vi "ModuloTeste.vi"(0 "IA State Input":T3 {"enemy_robots"."Agentes Disponíveis" format="%#_13g"; "our_robots"."Agentes Disponíveis" format="%#_13g"}, 1 "atacando ao contrário?":bool=TRUE, 3 "test module":T1) -> (14 "IA State Output":T3 {"enemy_robots"."Agentes Disponíveis" format="%#_13g"; "our_robots"."Agentes Disponíveis" format="%#_13g"}, 15 "ball":dbl(graph), 17 "Robot":dbl(graph))   [LabVIEW 2018]
uses:
  Core/AI Input.ctl
  Core/AI Robot.ctl
  Functions Enum.ctl
  AttackerStates.ctl
  Path Planning/RRT/PathDests.ctl
  Path Planning/RRT/PathDest.ctl
  Core/AI Ball.ctl
  Core/Field Size.ctl
  Core/AI Judge.ctl
  Command Enum.ctl
  Util/Events/Events.ctl
  Test/TestModule.ctl
  Util/Select None or Robot.ctl
  <vilib>/Analysis/_algsub.llb/Real Vector Norm.vi
  <vilib>/Analysis/NI_AALPro.lvlib
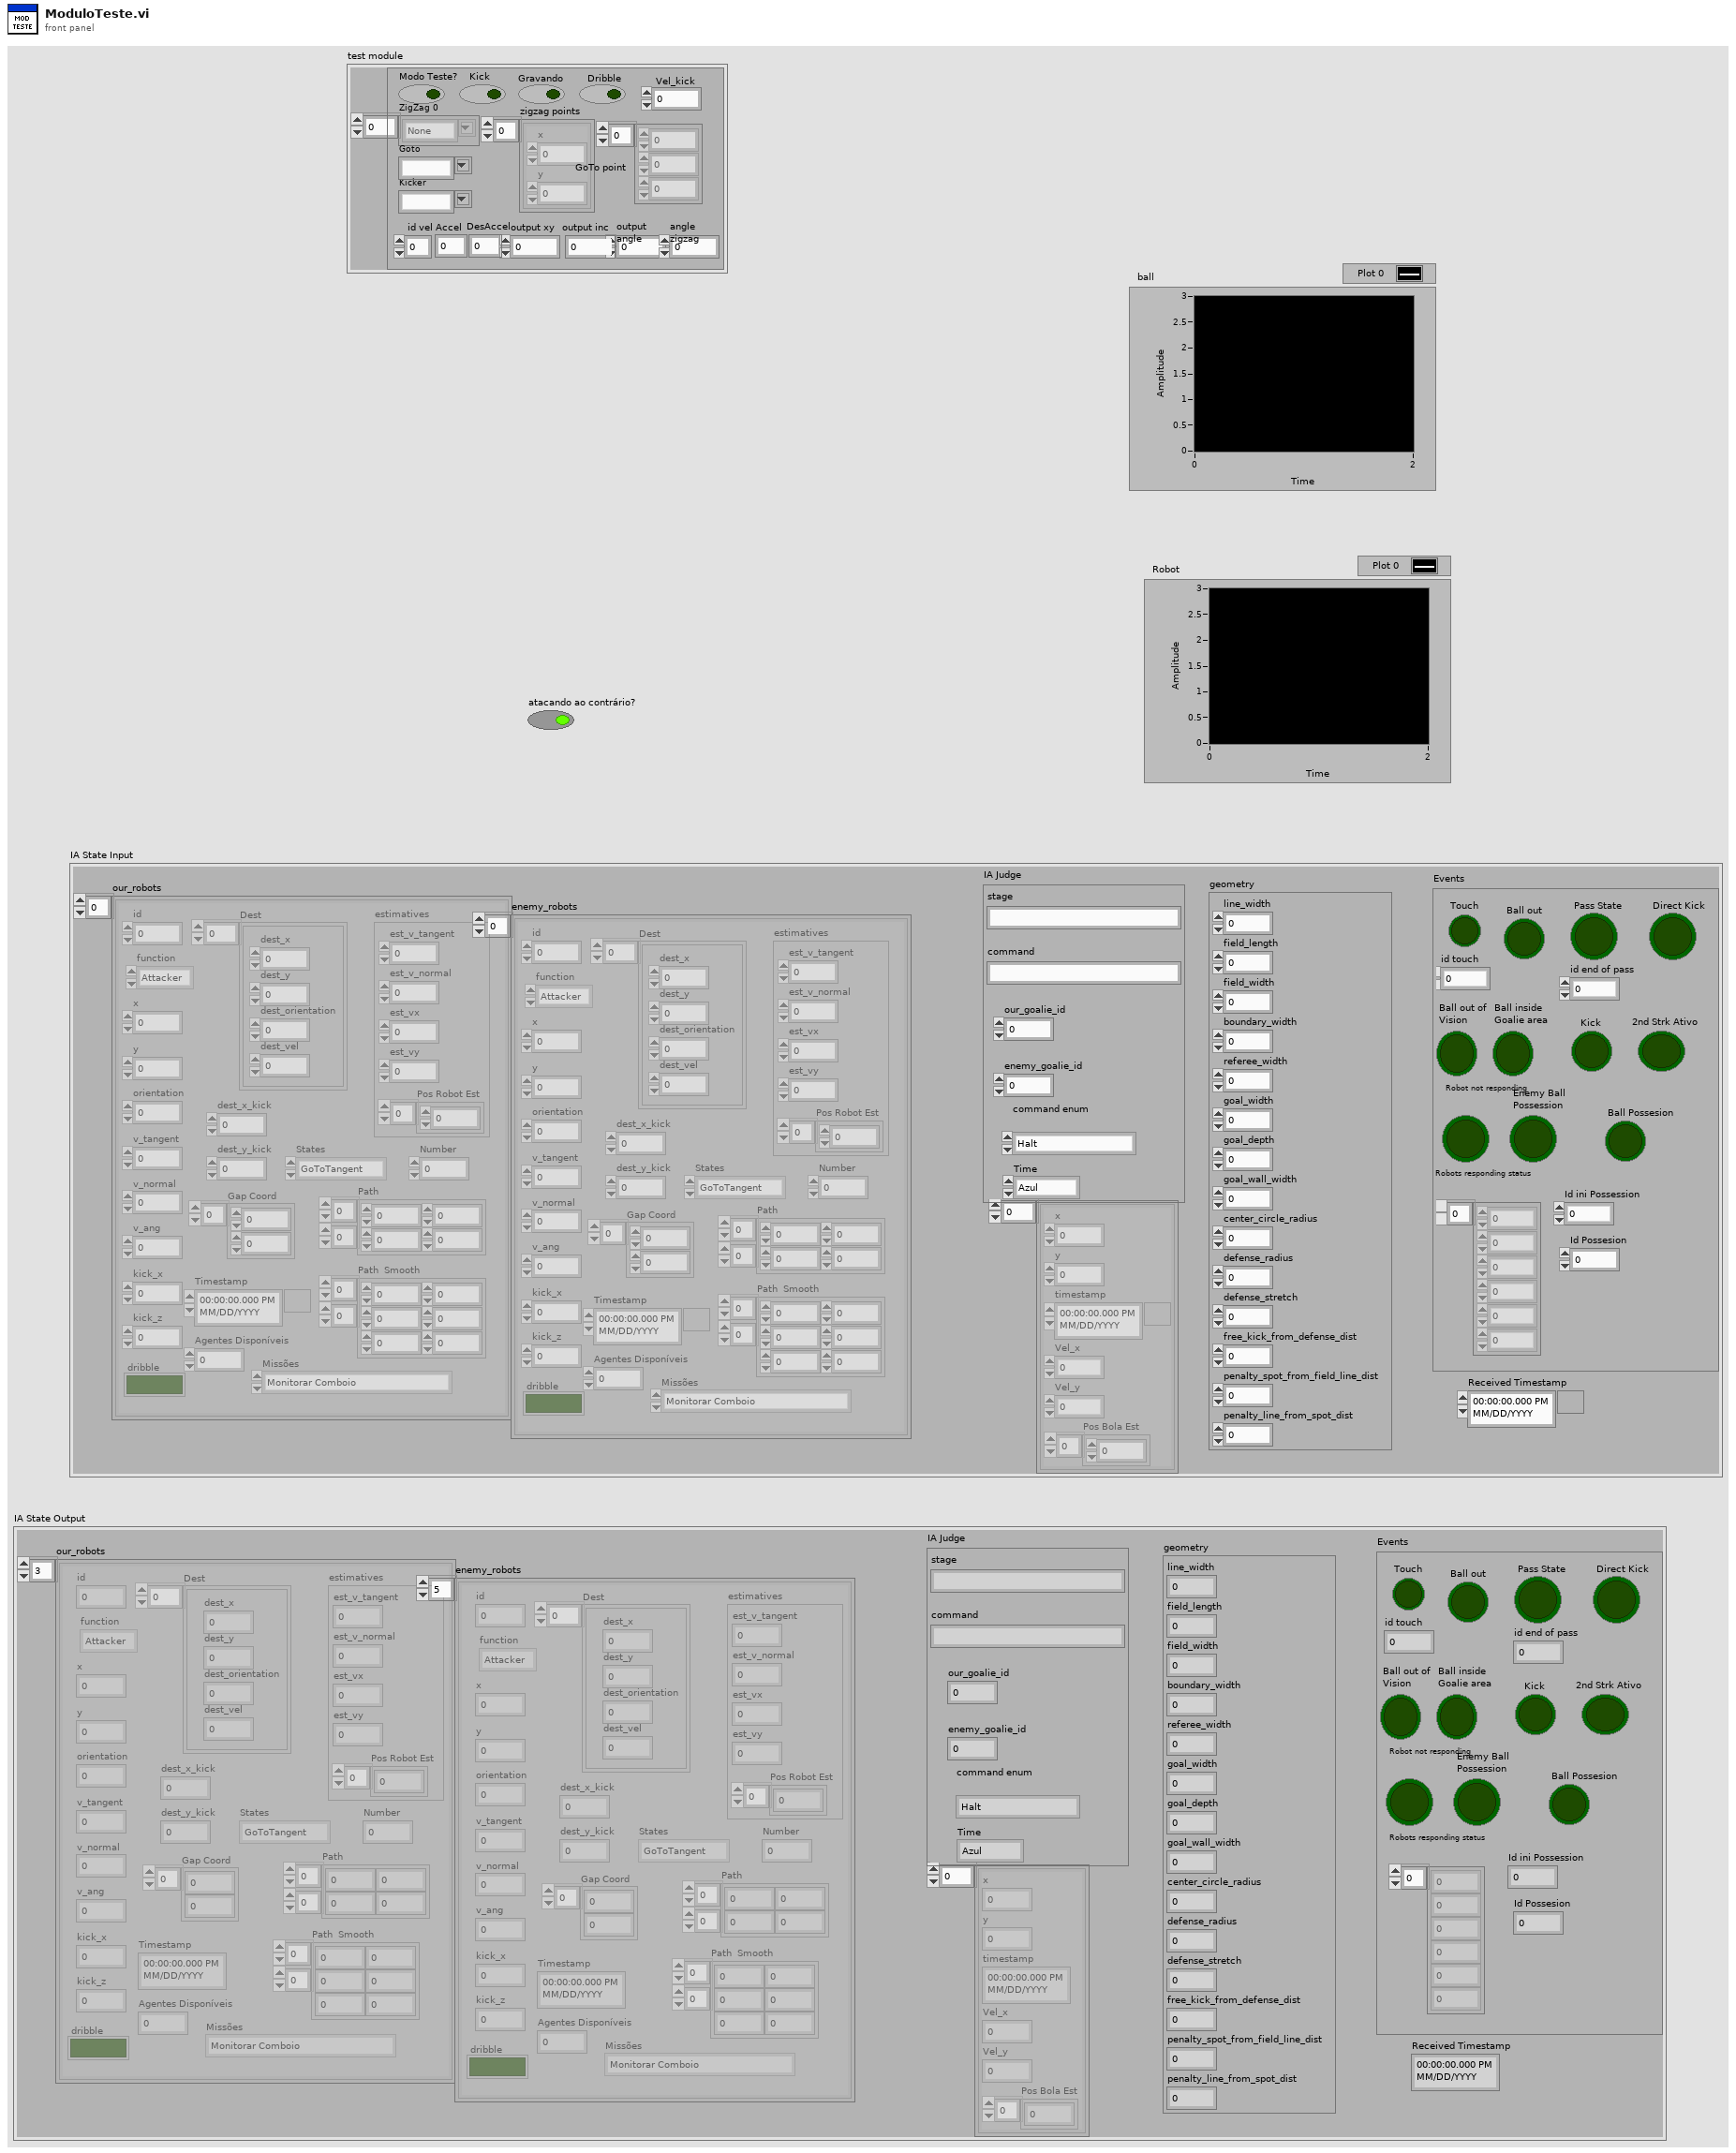
[diagram p1: front panel]
types:
  T1 = typedef "TestModule.ctl" = cluster{"Goto":T2, "ZigZag 0":T2[], "Kicker":T2, "Vel_kick":dbl, "Kick":bool, "Modo Teste?":bool, "GoTo point":dbl[], "zigzag points":cluster{"x":dbl, "y":dbl}[], " id vel":u32, "Dribble":bool, "Gravando":bool, "output xy":dbl, "output\nangle":dbl, "angle\nzigzag":dbl, "output inc":dbl, "Accel":dbl, "DesAccel":dbl}
  T2 = typedef "Select None or Robot.ctl" = string
  T3 = typedef "AI Input.ctl" = cluster{"our_robots":T4[], "enemy_robots":T4[], "balls":T9[], "geometry":T10, "IA Judge":T11, "Received Timestamp":timestamp, "Events":T13}
  T4 = typedef "AI Robot.ctl" = cluster{"id":u32, "function":T5, "x":dbl, "y":dbl, "orientation":dbl, "v_tangent":dbl, "v_normal":dbl, "v_ang":dbl, "kick_x":dbl, "kick_z":dbl, "dribble":bool, "Timestamp":timestamp, "estimatives":cluster{"est_v_tangent":dbl, "est_v_normal":dbl, "est_vx":dbl, "est_vy":dbl, "Pos Robot Est":dbl[]}, "dest_x_kick":dbl, "dest_y_kick":dbl, "Gap Coord":dbl[], "States":T6, "Path ":dbl[][], "Path  Smooth":dbl[][], "Dest":T7, "Missões ":enum16{"Monitorar Comboio", "Realizar Segurança de Retaguarda", "Vigiar Área", "Reconhecimento de Área"}, "Agentes Disponíveis":dbl, "Number":dbl}
  T5 = typedef "Functions Enum.ctl" = enum16{"None", "Vigia", "2nd Striker", "Attacker", "Goalie", "Defender", "Striker", "Goto 0", "Dummy", "Kicker", "ZigZag 0", "ZigZag 1", "ZigZag 2", "ZigZag 3", "ZigZag 4", "ZigZag 5", "ZigZag 6", "ZigZag 7", "ZigZag 8", ""}
  T6 = typedef "AttackerStates.ctl" = enum16{"Pass", "GoToTangent", "BallGetting", "GoToKick", ""}
  T7 = typedef "PathDests.ctl" = T8[]
  T8 = typedef "PathDest.ctl" = cluster{"dest_x":dbl, "dest_y":dbl, "dest_orientation":dbl, "dest_vel":dbl}
  T9 = typedef "AI Ball.ctl" = cluster{"x":dbl, "y":dbl, "timestamp":timestamp, "Vel_x":dbl, "Vel_y":dbl, "Pos Bola Est":dbl[]}
  T10 = typedef "Field Size.ctl" = cluster{"line_width":u32, "field_length":u32, "field_width":u32, "boundary_width":u32, "referee_width":u32, "goal_width":u32, "goal_depth":u32, "goal_wall_width":u32, "center_circle_radius":u32, "defense_radius":u32, "defense_stretch":u32, "free_kick_from_defense_dist":u32, "penalty_spot_from_field_line_dist":u32, "penalty_line_from_spot_dist":u32}
  T11 = typedef "AI Judge.ctl" = cluster{"stage":string, "command":string, "our_goalie_id":dbl, "enemy_goalie_id":dbl, "command enum":T12, "Time":enum16{"Azul", "Amarelo"}}
  T12 = typedef "Command Enum.ctl" = enum16{"Halt", "Stop", "Force Start", "PKA Normal Start", "Prepare Kickoff Ally", "PKE Normal Start", "Prepare Kickoff Enemy", "Prepare Penalty Ally", "PPA Normal Start", "Prepare Penalty Enemy", "PPE Normal Start", "Direct Free Enemy", "Direct Free Ally", "Indirect Free Enemy", "Indirect Free Ally", "Timeout Enemy", "Timeout Ally", "Goal Enemy", "Goal Ally", "Ball Placement Enemy", "Ball Placement Ally", "Normal Half Time", "Extra Time Break", "Extra Half Time", "None", "Post Game"}
  T13 = typedef "Events.ctl" = cluster{"Touch":bool, "Ball out":bool, "id touch":dbl, "Ball out of \nVision":bool, "Ball inside \nGoalie area":bool, "Robot not responding":bool, "Robots responding status":dbl[], "Enemy Ball \nPossession":bool, "Pass State":bool, "id end of pass":dbl, "Kick":bool, "Id ini Possession":dbl, "Ball Possesion":bool, "Id Possesion":dbl, "Direct Kick":bool, "2nd Strk Ativo":bool}
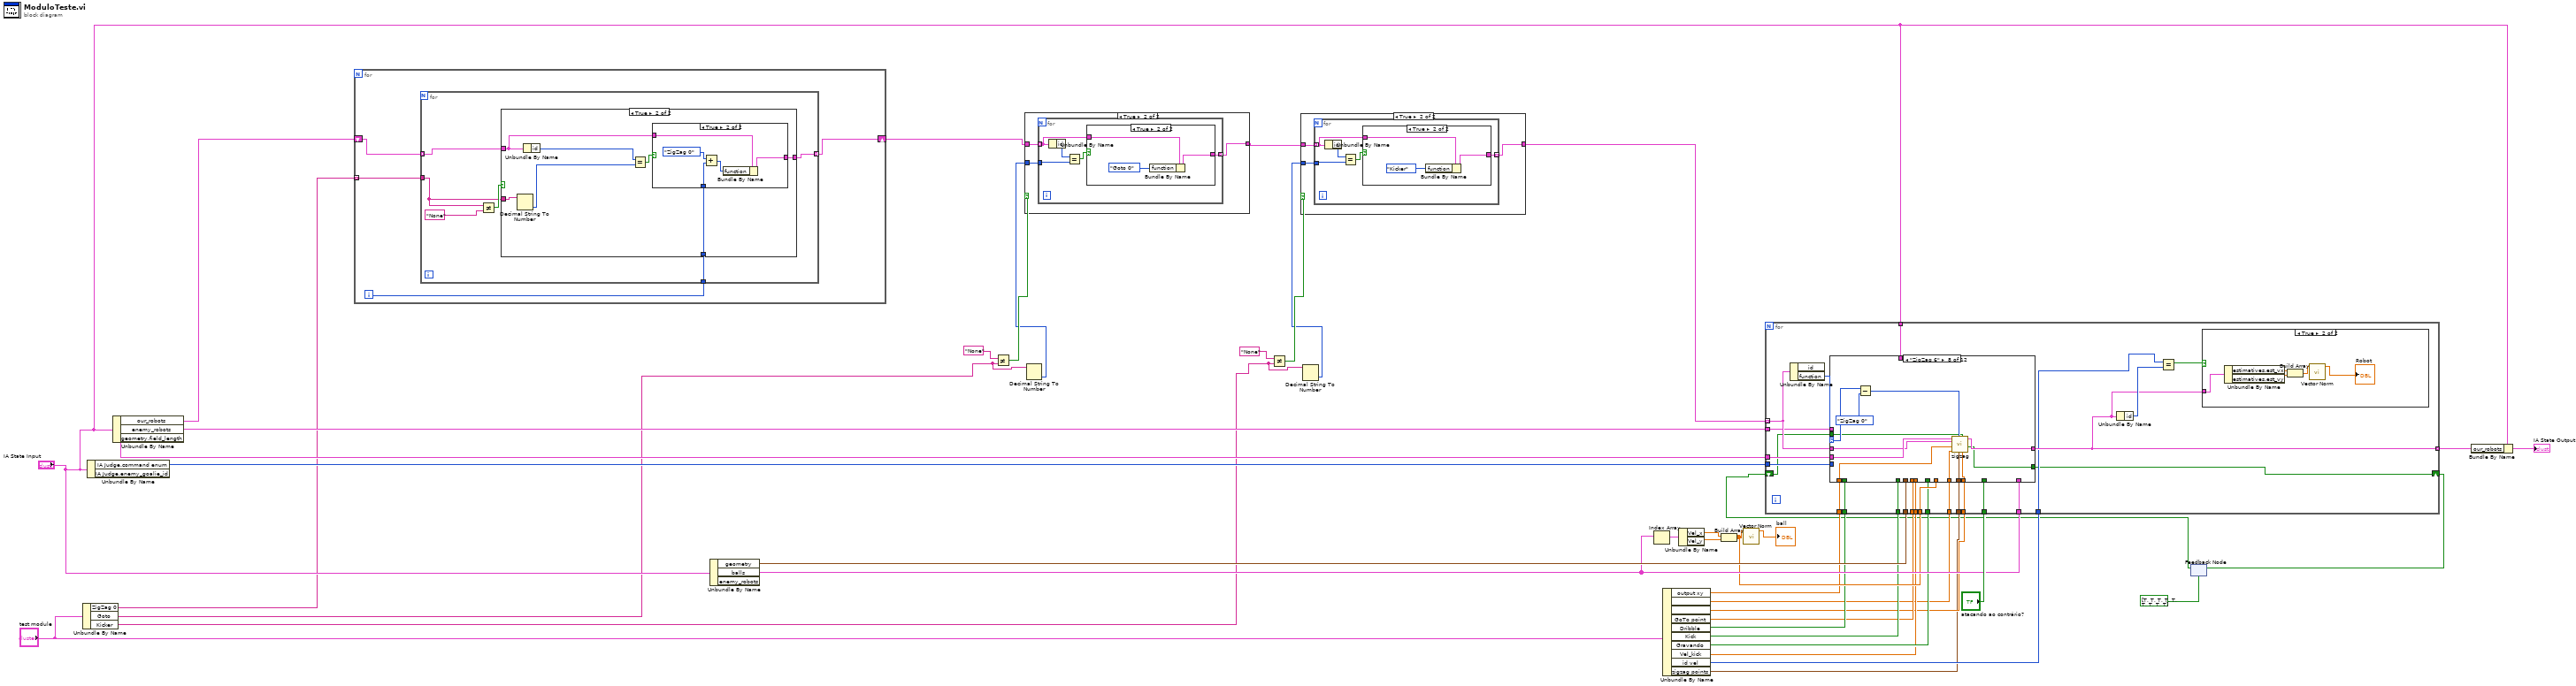
[diagram p0: block diagram]
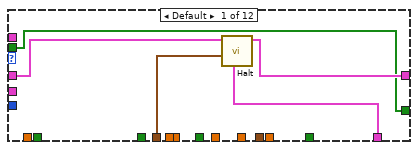
[diagram p9: hidden frame]
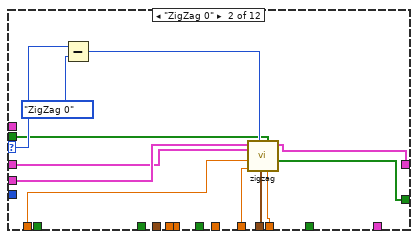
[diagram p10: hidden frame]
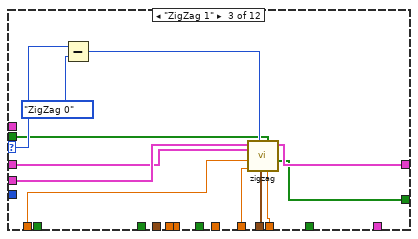
[diagram p11: hidden frame]
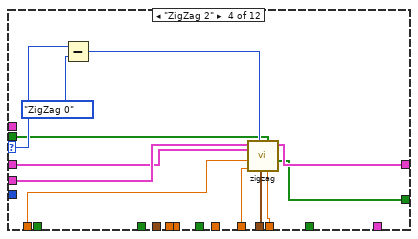
[diagram p12: hidden frame]
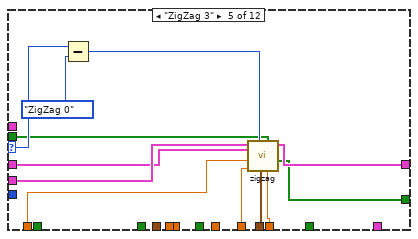
[diagram p13: hidden frame]
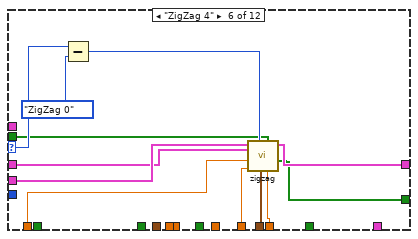
[diagram p14: hidden frame]
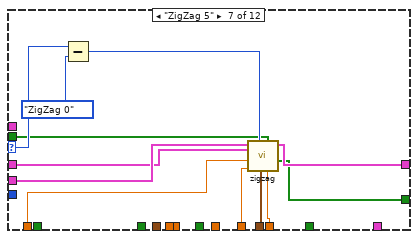
[diagram p15: hidden frame]
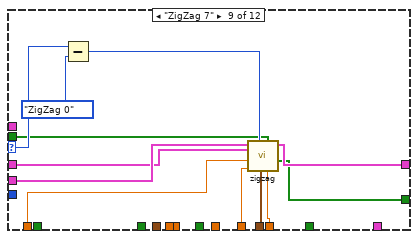
[diagram p16: hidden frame]
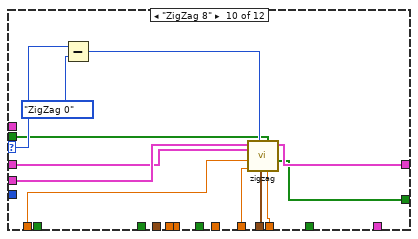
[diagram p17: hidden frame]
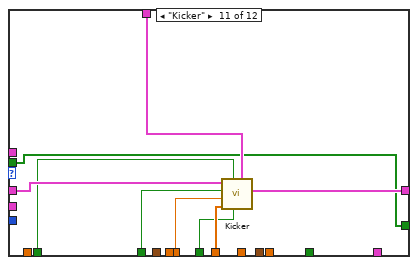
[diagram p18: hidden frame]
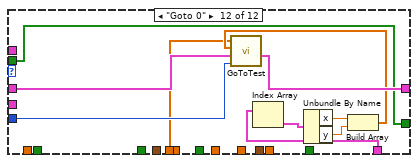
[diagram p19: hidden frame]
diagram:
  n1 = Unbundle By Name("test module") -> ("ZigZag 0"=w4:T2[], "Goto"=w17:T2, "Kicker"=w16:T2)
  n2 = Unbundle By Name("IA State Input") -> ("IA Judge.command enum"=w40:T12)  [unwired: 1 out]
  n3 = Unbundle By Name("IA State Input") -> ("our_robots"=w34:T4[], "enemy_robots"=w36:T4[])  [unwired: 1 out]
  n4 = for {
    tunnel: w4 -> [w43] mode=indexing
    shift-right: [w41] -> w31
    shift-left: w34 -> [w44]
    i -> [w42]
    n5 = for {
      tunnel: w43 -> [w46]
      tunnel: w42 -> [w45]
      tunnel: w44 -> [w49] mode=indexing
      tunnel: [w50] -> w41 mode=indexing
      n6 = Not Equal?(x=w46, y="None" ("x")) -> (x != y?=w47:bool)
      n7 = case shown="True" w47 {
        tunnel: [w51 w56] -> w50
        tunnel: w49 -> [w51 w55]
        tunnel: w46 -> [_ w54]
        tunnel: w45 -> [_ w52]
        frame False {
        }
        frame True {
          n8 = Decimal String To Number(string=w54) -> (number=w53:i32)  [unwired: 2 in, 1 out]
          n9 = Unbundle By Name(w55) -> ("id"=w58:u32)
          n10 = Equal?(x=w58, y=w53) -> (x = y?=w57:bool)
          n11 = case shown="True" w57 {
            tunnel: [w59 w64] -> w56
            tunnel: w55 -> [w59 w63]
            tunnel: w52 -> [_ w60]
            frame False {
            }
            frame True {
              n12 = Add(x=Functions_Enum."ZigZag 0" ("function"), y=w60) -> (x+y=w61:i32)
              n13 = Bundle By Name(cluster=w63, "function"=w61) -> (w64:T4)
            }
          }
        }
      }
    }
  }
  n14 = Unbundle By Name("IA State Input") -> ("geometry"=w37:T10, "balls"=w24:T9[])  [unwired: 1 out]
  n15 = Not Equal?(x="None", y=w17) -> (x != y?=w33:bool)
  n16 = Decimal String To Number(string=w17) -> (number=w30:i32)  [unwired: 2 in, 1 out]
  n17 = case shown="True" w33 {
    tunnel: w30 -> [_ w68]
    tunnel: [w65 w67] -> w26
    tunnel: w31 -> [w65 w66]
    frame False {
    }
    frame True {
      n18 = for {
        tunnel: w68 -> [w72]
        tunnel: [w70] -> w67 mode=indexing
        tunnel: w66 -> [w69] mode=indexing
        n19 = Unbundle By Name(w69) -> ("id"=w73:u32)
        n20 = Equal?(x=w73, y=w72) -> (x = y?=w71:bool)
        n21 = case shown="True" w71 {
          tunnel: [w74 w77] -> w70
          tunnel: w69 -> [w74 w75]
          frame False {
          }
          frame True {
            n22 = Bundle By Name(cluster=w75, "function"=Functions_Enum."Goto 0") -> (w77:T4)
          }
        }
      }
    }
  }
  n23 = Not Equal?(x="None", y=w16) -> (x != y?=w29:bool)
  n24 = Decimal String To Number(string=w16) -> (number=w27:i32)  [unwired: 2 in, 1 out]
  n25 = case shown="True" w29 {
    tunnel: w27 -> [_ w81]
    tunnel: [w78 w80] -> w25
    tunnel: w26 -> [w78 w79]
    frame False {
    }
    frame True {
      n26 = for {
        tunnel: w81 -> [w85]
        tunnel: [w83] -> w80 mode=indexing
        tunnel: w79 -> [w82] mode=indexing
        n27 = Unbundle By Name(w82) -> ("id"=w86:u32)
        n28 = Equal?(x=w86, y=w85) -> (x = y?=w84:bool)
        n29 = case shown="True" w84 {
          tunnel: [w87 w90] -> w83
          tunnel: w82 -> [w87 w88]
          frame False {
          }
          frame True {
            n30 = Bundle By Name(cluster=w88, "function"=Functions_Enum."Kicker") -> (w90:T4)
          }
        }
      }
    }
  }
  n31 = Index Array(array=w24) -> (element=w23:T9)  [unwired: 1 in]
  n32 = Unbundle By Name("test module") -> ("output xy"=w8:dbl, "output\nangle"=w7:dbl, "angle\nzigzag"=w6:dbl, "GoTo point"=w9:dbl[], "Dribble"=w14:bool, "Kick"=w13:bool, "Gravando"=w12:bool, "Vel_kick"=w11:dbl, "id vel"=w10:u32, "zigzag points"=w5:cluster{"x":dbl, "y":dbl}[])
  n33 = Unbundle By Name(w23) -> ("Vel_x"=w22:dbl, "Vel_y"=w21:dbl)
  n34 = Build Array(w22, w21) -> (w19:dbl[])
  n35 = call-poly <vilib>:"Vector Norm.vi"("Input Vector"=w19) -> ("norm"=→"ball":dbl)  [unwired: 9 in, 1 out]
  n36 = feedback #1(bool[] [TRUE, TRUE, TRUE, TRUE, TRUE, TRUE, TRUE, TRUE, TRUE]) -> (w1:bool[])
  n37 = for {
    tunnel: w25 -> [w114] mode=indexing
    tunnel: [w105] -> w39 mode=indexing
    tunnel: w40 -> [w113]
    tunnel: "IA State Input" -> [w112]
    tunnel: w37 -> [w111]
    tunnel: w24 -> [w110]
    tunnel: w36 -> [w109]
    tunnel: "atacando ao contrário?" -> [w108]
    tunnel: w5 -> [w104]
    tunnel: w19 -> [w103]
    tunnel: "IA State Input" -> [w102]
    tunnel: w14 -> [w101]
    tunnel: w13 -> [w100]
    tunnel: w12 -> [w99]
    tunnel: w11 -> [w98]
    tunnel: w10 -> [w97]
    tunnel: w9 -> [w96]
    tunnel: w8 -> [w95]
    tunnel: w7 -> [w94]
    tunnel: w6 -> [w93]
    shift-right: [w91] -> w3
    shift-left: w1 -> [w92]
    n38 = Unbundle By Name(w114) -> ("function"=w115:T5)  [unwired: 1 out]
    n39 = case shown="\"ZigZag 6\"" w115 {
      selector: w115 -> [_ w130 w142 w154 w166 w178 w190 w202 w214 w226 _ _]
      tunnel: w114 -> [w125 w135 w147 w159 w171 w183 w195 w207 w219 w231 w241 w252]
      tunnel: [w124 w137 w149 w161 w173 w185 w197 w209 w221 w233 w242 w251] -> w105
      tunnel: w113 -> [_ _ _ _ _ _ _ _ _ _ _ w250]
      tunnel: w112 -> [_ w136 w148 w160 w172 w184 w196 w208 w220 w232 _ _]
      tunnel: w111 -> [w123 _ _ _ _ _ _ _ _ _ _ _]
      tunnel: w110 -> [w122 _ _ _ _ _ _ _ _ _ _ w249]
      tunnel: w109 -> [_ _ _ _ _ _ _ _ _ _ _ _]
      tunnel: w108 -> [_ _ _ _ _ _ _ _ _ _ _ _]
      tunnel: w104 -> [_ w134 w146 w158 w170 w182 w194 w206 w218 w230 _ _]
      tunnel: w103 -> [_ _ _ _ _ _ _ _ _ _ w240 _]
      tunnel: w102 -> [_ _ _ _ _ _ _ _ _ _ w239 _]
      tunnel: w101 -> [_ _ _ _ _ _ _ _ _ _ w238 _]
      tunnel: w100 -> [_ _ _ _ _ _ _ _ _ _ w237 _]
      tunnel: w99 -> [_ _ _ _ _ _ _ _ _ _ w236 _]
      tunnel: w98 -> [_ _ _ _ _ _ _ _ _ _ w235 _]
      tunnel: w96 -> [_ _ _ _ _ _ _ _ _ _ _ w244]
      tunnel: w95 -> [_ w133 w145 w157 w169 w181 w193 w205 w217 w229 _ _]
      tunnel: w94 -> [_ w132 w144 w156 w168 w180 w192 w204 w216 w228 _ _]
      tunnel: w93 -> [_ w131 w143 w155 w167 w179 w191 w203 w215 w227 _ _]
      tunnel: w92 -> [w121 w127 w139 w151 w163 w175 w187 w199 w211 w223 w234 w243]
      tunnel: [w121 w126 w138 w150 w162 w174 w186 w198 w210 w222 w234 w243] -> w91
      frame Default {
        n40 = call "Halt.vi"("balls"=w122, "Field Size in"=w123, "Robot in"=w125) -> ("Robot out"=w124:T4)  [unwired: 8 in]
      }
      frame "ZigZag 0" {
        n41 = Subtract(x=w130, y=Functions_Enum."ZigZag 0") -> (x-y=w128:u16)
        n42 = call "zigzag.vi"("angulo"=w131, "Change point by ID"=w127, "points 3"=w134, "ZigZag Number"=w128, "output angle"=w132, "output xy"=w133, "Current Robot"=w135, "Al Input"=w136) -> ("output array"=w126:bool[], "Output Robot"=w137:T4)  [unwired: 1 in, 1 out]
      }
      frame "ZigZag 1" {
        n43 = Subtract(x=w142, y=Functions_Enum."ZigZag 0") -> (x-y=w140:u16)
        n44 = call "zigzag.vi"("angulo"=w143, "Change point by ID"=w139, "points 3"=w146, "ZigZag Number"=w140, "output angle"=w144, "output xy"=w145, "Current Robot"=w147, "Al Input"=w148) -> ("output array"=w138:bool[], "Output Robot"=w149:T4)  [unwired: 1 in, 1 out]
      }
      frame "ZigZag 2" {
        n45 = Subtract(x=w154, y=Functions_Enum."ZigZag 0") -> (x-y=w152:u16)
        n46 = call "zigzag.vi"("angulo"=w155, "Change point by ID"=w151, "points 3"=w158, "ZigZag Number"=w152, "output angle"=w156, "output xy"=w157, "Current Robot"=w159, "Al Input"=w160) -> ("output array"=w150:bool[], "Output Robot"=w161:T4)  [unwired: 1 in, 1 out]
      }
      frame "ZigZag 3" {
        n47 = Subtract(x=w166, y=Functions_Enum."ZigZag 0") -> (x-y=w164:u16)
        n48 = call "zigzag.vi"("angulo"=w167, "Change point by ID"=w163, "points 3"=w170, "ZigZag Number"=w164, "output angle"=w168, "output xy"=w169, "Current Robot"=w171, "Al Input"=w172) -> ("output array"=w162:bool[], "Output Robot"=w173:T4)  [unwired: 1 in, 1 out]
      }
      frame "ZigZag 4" {
        n49 = Subtract(x=w178, y=Functions_Enum."ZigZag 0") -> (x-y=w176:u16)
        n50 = call "zigzag.vi"("angulo"=w179, "Change point by ID"=w175, "points 3"=w182, "ZigZag Number"=w176, "output angle"=w180, "output xy"=w181, "Current Robot"=w183, "Al Input"=w184) -> ("output array"=w174:bool[], "Output Robot"=w185:T4)  [unwired: 1 in, 1 out]
      }
      frame "ZigZag 5" {
        n51 = Subtract(x=w190, y=Functions_Enum."ZigZag 0") -> (x-y=w188:u16)
        n52 = call "zigzag.vi"("angulo"=w191, "Change point by ID"=w187, "points 3"=w194, "ZigZag Number"=w188, "output angle"=w192, "output xy"=w193, "Current Robot"=w195, "Al Input"=w196) -> ("output array"=w186:bool[], "Output Robot"=w197:T4)  [unwired: 1 in, 1 out]
      }
      frame "ZigZag 6" {
        n53 = Subtract(x=w202, y=Functions_Enum."ZigZag 0") -> (x-y=w200:u16)
        n54 = call "zigzag.vi"("angulo"=w203, "Change point by ID"=w199, "points 3"=w206, "ZigZag Number"=w200, "output angle"=w204, "output xy"=w205, "Current Robot"=w207, "Al Input"=w208) -> ("output array"=w198:bool[], "Output Robot"=w209:T4)  [unwired: 1 in, 1 out]
      }
      frame "ZigZag 7" {
        n55 = Subtract(x=w214, y=Functions_Enum."ZigZag 0") -> (x-y=w212:u16)
        n56 = call "zigzag.vi"("angulo"=w215, "Change point by ID"=w211, "points 3"=w218, "ZigZag Number"=w212, "output angle"=w216, "output xy"=w217, "Current Robot"=w219, "Al Input"=w220) -> ("output array"=w210:bool[], "Output Robot"=w221:T4)  [unwired: 1 in, 1 out]
      }
      frame "ZigZag 8" {
        n57 = Subtract(x=w226, y=Functions_Enum."ZigZag 0") -> (x-y=w224:u16)
        n58 = call "zigzag.vi"("angulo"=w227, "Change point by ID"=w223, "points 3"=w230, "ZigZag Number"=w224, "output angle"=w228, "output xy"=w229, "Current Robot"=w231, "Al Input"=w232) -> ("output array"=w222:bool[], "Output Robot"=w233:T4)  [unwired: 1 in, 1 out]
      }
      frame "Kicker" {
        n59 = call "Kicker.vi"("IA State Input"=w239, "gravar"=w236, "Dribble"=w238, "Ball velocity"=w240, "Vel_kick"=w235, "Kick?"=w237, "Robot in"=w241) -> ("output cluster"=w242:T4)  [unwired: 4 in]
      }
      frame "Goto 0" {
        n60 = Index Array(array=w249) -> (element=w248:T9)  [unwired: 1 in]
        n61 = Unbundle By Name(w248) -> ("x"=w247:dbl, "y"=w246:dbl)
        n62 = Build Array(w247, w246) -> (w245:dbl[])
        n63 = call "GoToTest.vi"("command\nenum"=w250, "Robot In"=w252, "Ball"=w245, "GoTo point"=w244) -> ("Robot Out"=w251:T4)  [unwired: 7 in]
      }
    }
    n64 = Unbundle By Name(w105) -> ("id"=w107:u32)
    n65 = Equal?(x=w97, y=w107) -> (x = y?=w106:bool)
    n66 = case shown="True" w106 {
      tunnel: w105 -> [_ w120]
      frame False {
      }
      frame True {
        n67 = Unbundle By Name(w120) -> ("estimatives.est_vx"=w119:dbl, "estimatives.est_vy"=w118:dbl)
        n68 = Build Array(w119, w118) -> (w117:dbl[])
        n69 = call-poly <vilib>:"Vector Norm.vi"("Input Vector"=w117) -> ("norm"=→"Robot":dbl)  [unwired: 9 in, 1 out]
      }
    }
  }
  n70 = feedback-in #1(w3) -> ()
  n71 = Bundle By Name(cluster="IA State Input", "our_robots"=w39) -> (→"IA State Output":T3)
